vi "PeriodTimeToSQLDateTime.vi"(8 "day":i32, 9 "Month":i32, 11 "string":string) -> (0 "StingDate":string, 1 "SQLDatetime2":string, 3 "SQLDateTime1":string, 4 "Period(M)":dbl)   [LabVIEW 2012]
uses:
  <vilib>/Utility/miscctls.llb/LVDateTimeRec.ctl
panel:
  in  "date time rec":T1
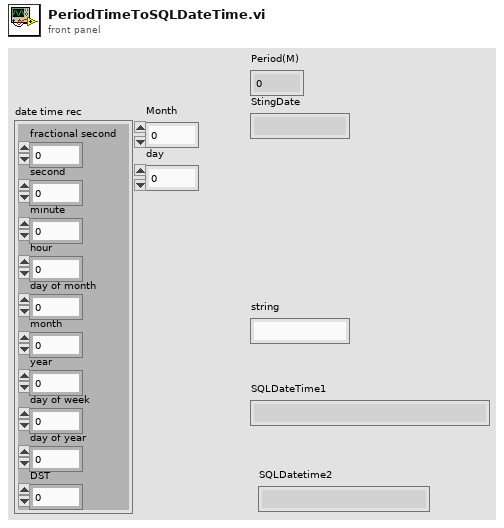
[diagram p1: front panel]
types:
  T1 = typedef "LVDateTimeRec.ctl" = cluster{"fractional second":dbl, "second":i32, "minute":i32, "hour":i32, "day of month":i32, "month":i32, "year":i32, "day of week":i32, "day of year":i32, "DST":i32}
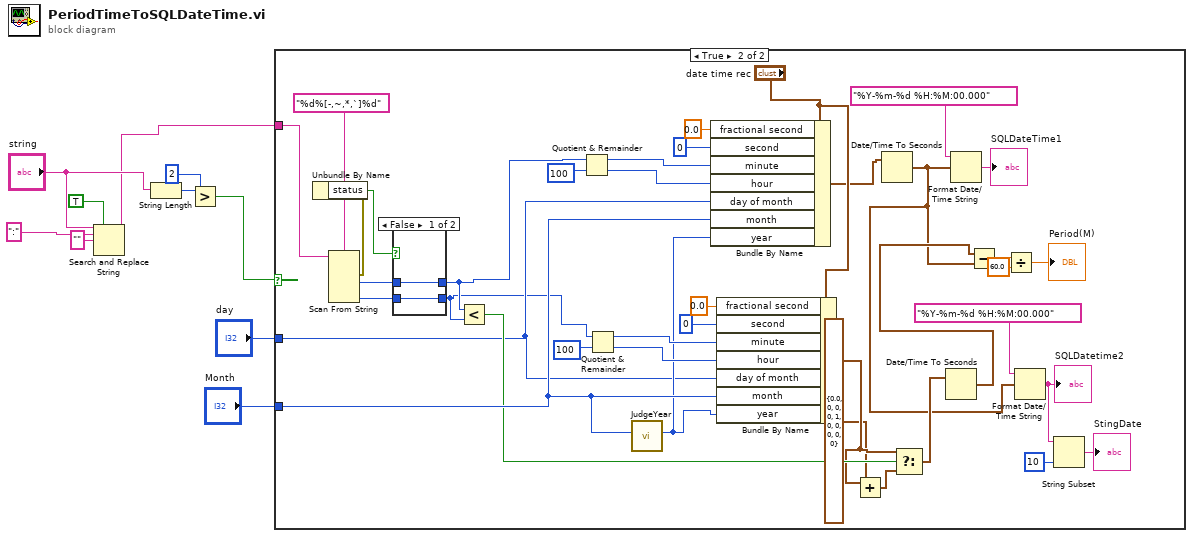
[diagram p0: block diagram]
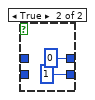
[diagram p3: hidden frame]
diagram:
  n1 = Search and Replace String(replace all?=TRUE ("replace all? (F)"), input string="string", search string=":", replace string="" ("replace string (\"\")")) -> (result string=w2:string)  [unwired: 4 in, 3 out]
  n2 = String Length(string="string") -> (length=w8:i32)
  n3 = Greater?(x=w8, y=2) -> (0:w6:bool)
  n4 = case shown="True" w6 {
    tunnel: "day" -> [_ w22]
    tunnel: "Month" -> [_ w37]
    tunnel: w2 -> [_ w28]
    frame False {
    }
    frame True {
      n5 = Scan From String(format string="%d%[-,~,*,`]%d", input string=w28) -> (error out=w16:errorcluster, output 1=w14:i32, output 3=w11:i32)  [unwired: 6 in, 2 out]
      n6 = Unbundle By Name(w16) -> ("status"=w15:bool)
      n7 = case shown="False" w15 {
        tunnel: w14 -> [w50 _]
        tunnel: [w50 0] -> w13
        tunnel: [w51 1] -> w12
        tunnel: w11 -> [w51 _]
        frame False {
        }
        frame True {
        }
      }
      n8 = Less?(x=w13, y=w12) -> (x < y?=w23:bool)
      n9 = Quotient & Remainder(x=w13, y=100) -> (x-y*floor(x/y)=w46:i32, floor(x/y)=w45:i32)
      n10 = Quotient & Remainder(x=w12, y=100) -> (x-y*floor(x/y)=w41:i32, floor(x/y)=w40:i32)
      n11 = call "JudgeYear.vi"("DataMonth"=w37) -> ("DataYear"=w36:i32)  [unwired: 10 in]
      n12 = Bundle By Name(cluster="date time rec", "fractional second"=0.0, "second"=0, "minute"=w46, "hour"=w45, "day of month"=w22, "month"=w37, "year"=w36) -> (w35:T1)
      n13 = Bundle By Name(cluster="date time rec", "fractional second"=0.0, "second"=0, "minute"=w41, "hour"=w40, "day of month"=w22, "month"=w37, "year"=w36) -> (w20:T1)
      n14 = Add(x=w20, y=T1 {"fractional second"=0.0, "second"=0, "minute"=0, "hour"=0, "day of month"=1, "month"=0, "year"=0, "day of week"=0, "day of year"=0, "DST"=0}) -> (x+y=w19:T1)
      n15 = Date/Time To Seconds(2:w35) -> (0:w17:timestamp)  [unwired: 1 in]
      n16 = Select(t=w20, s=w23, f=w19) -> (s? t:f=w21:T1)
      n17 = Date/Time To Seconds(2:w21) -> (0:w27:timestamp)  [unwired: 1 in]
      n18 = Format Date/Time String(time format string (%c)="%Y-%m-%d %H:%M:00.000", seconds (now)=w17) -> (date/time string=→"SQLDateTime1":string)  [unwired: 1 in]
      n19 = Subtract(x=w27, y=w17) -> (x-y=w31:dbl)
      n20 = Divide(x=w31, y=60.0) -> (x/y=→"Period(M)":dbl)
      n21 = Format Date/Time String(time format string (%c)="%Y-%m-%d %H:%M:00.000", seconds (now)=w17) -> (date/time string=w26:string)  [unwired: 1 in]
      "SQLDatetime2" <- w26
      n22 = String Subset(string=w26, length (rest)=10 ("length (rest)")) -> (substring=→"StingDate":string)  [unwired: 1 in]
    }
  }
